vi "SetTriggerMode.vi"(9 "Trigger":refnum<vi>, 10 "ExposureMode":refnum<k24>, 11 "Digital in":refnum<vi>) -> ()   [LabVIEW 2018]
uses:
  D:/SVN/PM/sdk/AppSamples/LabVIEWSamples/trunk/Release/2018/Dependencies/PVCamNET.dll
  Dependencies/PVCamNET.dll
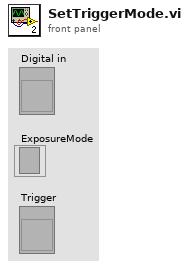
[diagram p1: front panel]
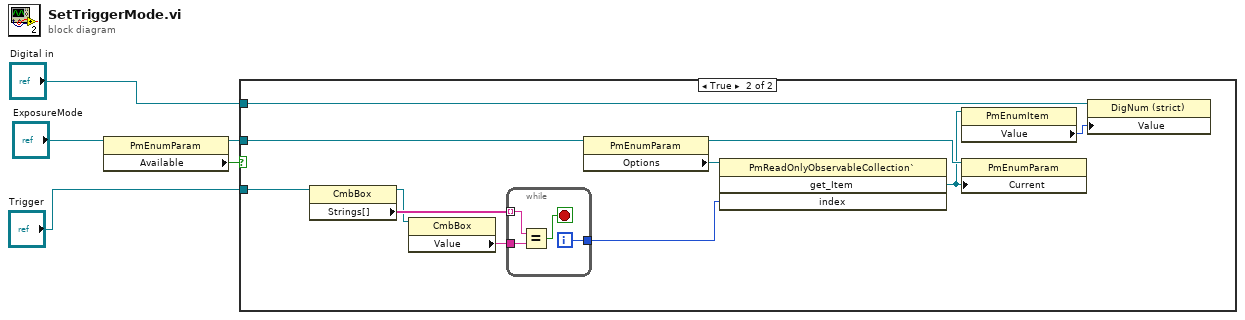
[diagram p0: block diagram]
diagram:
  n1 = property class="PmEnumParam"(reference="ExposureMode") -> (reference out=w4:refnum<k24>, "Available"=w3:bool)  [unwired: 1 in, 1 out]
  n2 = case shown="True" w3 {
    tunnel: w4 -> [_ w15]
    tunnel: "Digital in" -> [_ w9]
    tunnel: "Trigger" -> [_ w6]
    frame False {
    }
    frame True {
      n3 = property class="CmbBox"(reference=w6) -> (reference out=w8:refnum<vi>, "Strings[]"=w16:string[])  [unwired: 1 in, 1 out]
      n4 = property class="CmbBox"(reference=w8) -> ("Value"=w7:string)  [unwired: 1 in, 2 out]
      n5 = while {
        tunnel: w16 -> [w20] mode=indexing
        tunnel: [w18] -> w13
        tunnel: w7 -> [w17]
        i -> [w18]
        stop <- w19 stop-if-true
        n6 = Equal?(x=w20, y=w17) -> (x = y?=w19:bool)
      }
      n7 = property class="PmEnumParam"(reference=w15) -> (reference out=w12:refnum<k24>, "Options"=w14:refnum<k24>)  [unwired: 1 in, 1 out]
      n8 = invoke class="PmReadOnlyObservableCollection`" method="get_Item"(reference=w14, "index"=w13) -> ("get_Item"=w11:refnum<k24>)  [unwired: 2 in, 3 out]
      n9 = property class="PmEnumItem"(reference=w11) -> ("Value"=w10:i32)  [unwired: 1 in, 2 out]
      n10 = property class="PmEnumParam"(reference=w12, "Current"=w11) -> ()  [unwired: 1 in, 2 out]
      n11 = property class="DigNum (strict)"(reference=w9, "Value"=w10) -> ()  [unwired: 1 in, 2 out]
    }
  }
